vi "OE1022D_Configure Filter.vi"(5 "Low Pass Filter Slope (1: 12dB/oct)":u8(ring)=1 items=["6 dB/oct", "12 dB/oct", "18 db/oct", "24 dB/oct"], 7 "Time Constant (8: 100ms)":u8(ring)=9 items=["10 us", "30 us", "100 us", "300 us", "1 ms", "3 ms", "10 ms", "30 ms", "100 ms", "300 ms", "1 s", "3 s", "10 s", "30 s", "100 s", "300 s", "1 ks", "3 ks"], 8 "error in (no error)":errorcluster, 9 "Enable Sync Filter (F: Disable)":bool, 10 "OE1022D A/B":u8(ring) items=["Channel A", "Channel B"], 11 "VISA resource name":refnum<visa-resource-name>) -> (0 "error out":errorcluster, 3 "VISA resource name out":refnum<visa-resource-name>)   [LabVIEW 2014]
doc: "Configures the instrument's filter options.\n\n<B>Note:</B>\n\nThe Notch Filter is configured in <B>Configure Input Signal.vi</B>"
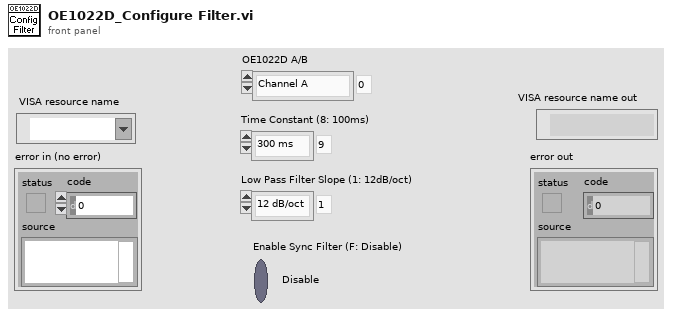
[diagram p1: front panel]
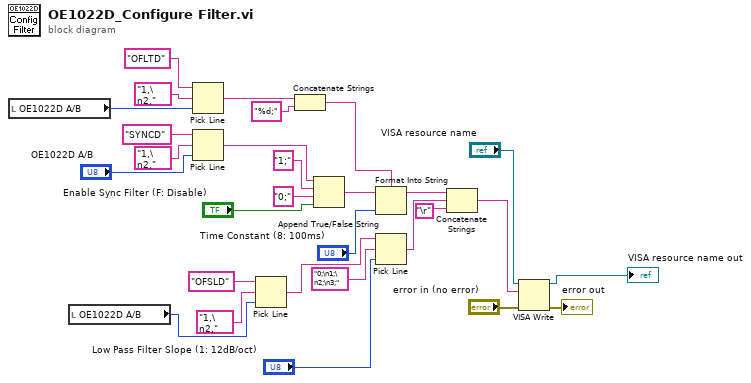
[diagram p0: block diagram]
diagram:
  n1 = local read "OE1022D A/B"() -> (w13:u8)
  n2 = local read "OE1022D A/B"() -> (w7:u8)
  n3 = Pick Line(string ("")="OFLTD", multi-line string="1,\n2,", line index=w13) -> (output string=w12:string)
  n4 = Pick Line(string ("")="SYNCD", multi-line string="1,\n2,", line index="OE1022D A/B") -> (output string=w16:string)
  n5 = Pick Line(string ("")="OFSLD", multi-line string="1,\n2,", line index=w7) -> (output string=w5:string)
  n6 = Concatenate Strings(w12, "%d;" ("format string")) -> (w10:string)
  n7 = Append True/False String(1:"Enable Sync Filter (F: Disable)", 2:"0;" ("false string"), 3:"1;" ("true string"), 4:w16) -> (0:w24:string)
  n8 = Format Into String(format string=w10, initial string=w24, "Time Constant (8: 100ms)") -> (resulting string=w3:string)  [unwired: 1 in, 1 out]
  n9 = Pick Line(string ("")=w5, multi-line string="0;\n1;\n2;\n3;", line index="Low Pass Filter Slope (1: 12dB/oct)") -> (output string=w2:string)
  n10 = Concatenate Strings(w3, w2, "\r") -> (w21:string)
  n11 = VISA Write(VISA resource name="VISA resource name", write buffer=w21, error in (no error)="error in (no error)") -> (VISA resource name out=→"VISA resource name out":refnum<visa-resource-name>, error out=→"error out":errorcluster)  [unwired: 1 out]
